vi "date_txt.vi"() -> ()   [LabVIEW 2017]
panel:
  in  "date_txt":dbl
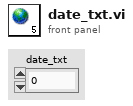
[diagram p1: front panel]
diagram:
